vi "load csv taglist.vi"(10 "cfg file path":path) -> (2 "ok?":bool, 3 "tags":refnum<class "tag descriptor.lvclass">[](array[class]))   [LabVIEW 2013, in "PL Framework Configuration Tool.lvlib" / "EngineTags.lvclass"]
uses:
  EngineTags.lvclass
  <vilib>/NI/Tag Bus/tag/tag descriptor.lvclass
  <vilib>/NI/Tag Bus/tag/count types.vi
  <vilib>/NI/Tag Bus/tag/index to type.vi
  Robust CSV/Robust CSV.lvlib
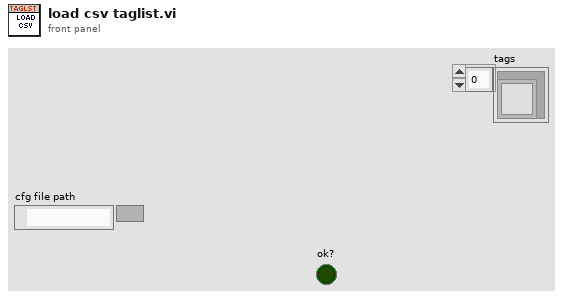
[diagram p1: front panel]
types:
  T1 = enum16{"open", "replace", "create", "open or create", "replace or create", "replace or create with confirmation"}
  T2 = typedef "tag bus.lvlib/tag descriptor.lvclass/Data Type.ctl" = enum16{"Double", "Single", "I64", "I32", "I16", "I8", "U64", "U32", "U16", "U8", "Boolean", "String", "Array of Double", "Array of Single", "Array of I64", "Array of I32", "Array of I16", "Array of I8", "Array of U64", "Array of U32", "Array of U16", "Array of U8", "Array of Boolean", "Array of String"}
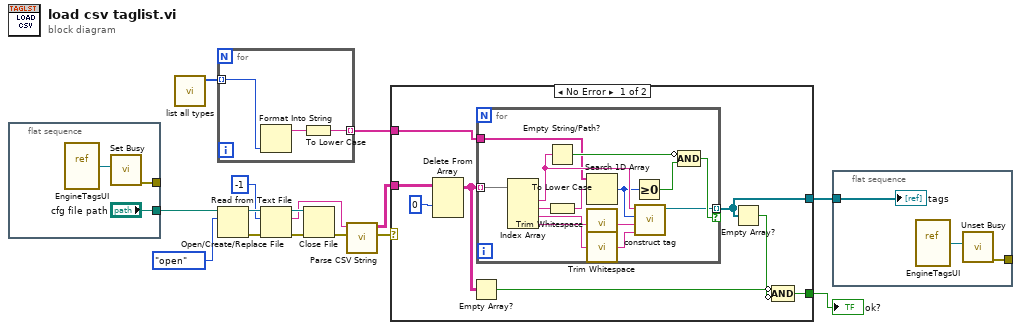
[diagram p0: block diagram]
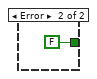
[diagram p2: hidden frame]
diagram:
  n1 = flat-sequence {
    tunnel: [w17] -> _
    tunnel: ["cfg file path"] -> w9
    frame #0 {
      n2 = vi-ref "EngineTagsUI.vi"() -> (w18:refnum<vi>)
      n3 = call <vilib>:"Set Busy.vi"("VI reference (current VI)"=w18) -> ("error out"=w17:errorcluster)  [unwired: 9 in, 1 out]
    }
  }
  n4 = call <vilib>:"list all types.vi"() -> ("all types"=w6:T2[])  [unwired: 11 in]
  n5 = for {
    tunnel: w6 -> [w21] mode=indexing
    tunnel: [w19] -> w5 mode=indexing
    n6 = Format Into String(w21) -> (resulting string=w20:string)  [unwired: 3 in, 1 out]
    n7 = To Lower Case(string=w20) -> (all lower case string=w19:string)
  }
  n8 = Open/Create/Replace File(file path (use dialog)=w9, operation (0:open)=T1."open") -> (refnum out=w13:refnum<file>, error out=w12:errorcluster)  [unwired: 4 in, 1 out]
  n9 = Read from Text File(file (use dialog)=w13, count=-1, error in=w12) -> (refnum out=w11:refnum<file>, text=w3:string, error out=w10:errorcluster)  [unwired: 1 in, 1 out]
  n10 = Close File(refnum=w11, error in=w10) -> (error out=w4:errorcluster)  [unwired: 1 out]
  n11 = call "Parse CSV String.vi"("error in"=w4, "CSV string"=w3) -> ("error out"=w1:errorcluster, "2-D array"=w2:string[][])  [unwired: 8 in]
  n12 = case shown="No Error" w1 {
    tunnel: w2 -> [w22 _]
    tunnel: [w26 _] -> w15
    tunnel: [w24 FALSE] -> w14
    tunnel: w5 -> [w23 _]
    frame No Error {
      n13 = Delete From Array(array=w22, index (row)=0) -> (array with subset deleted=w28:string[][])  [unwired: 2 in, 1 out]
      n14 = Empty Array?(array=w28) -> (empty?=w27:bool)
      n15 = for {
        tunnel: [w39] -> w26 mode=indexing if=w42
        tunnel: w28 -> [w30] mode=indexing
        tunnel: w23 -> [w33]
        n16 = Index Array(array=w30) -> (element #1=w36:string, element #2=w35:string, element #3=w37:string, element #4=w38:string)  [unwired: 4 in]
        n17 = Empty String/Path?(string/path=w36) -> (empty?=w43:bool)
        n18 = To Lower Case(string=w35) -> (all lower case string=w34:string)
        n19 = Search 1D Array(1D array=w33, element=w34) -> (index of element=w31:i32)  [unwired: 1 in]
        n20 = call <vilib>:"Trim Whitespace.vi"("string"=w38) -> ("trimmed string"=w41:string)  [unwired: 1 in]
        n21 = call <vilib>:"Trim Whitespace.vi"("string"=w37) -> ("trimmed string"=w40:string)  [unwired: 1 in]
        n22 = Greater Or Equal To 0?(x=w31) -> (x >= 0?=w32:bool)
        n23 = call <vilib>:"construct tag.vi"("raw default"=w40, "metadata"=w41, "data type"=w31, "name"=w36) -> ("system tag out"=w39:refnum<class "tag descriptor.lvclass">)  [unwired: 6 in, 1 out]
        n24 = Compound Arithmetic op=AND(invert w43, w32) -> (w42:bool)
      }
      n25 = Empty Array?(array=w26) -> (empty?=w25:bool)
      n26 = Compound Arithmetic op=AND(invert w27, invert w25) -> (w24:bool)
    }
    frame Error {
    }
  }
  "ok?" <- w14
  n27 = flat-sequence {
    tunnel: w15 -> [w45]
    tunnel: [w46] -> _
    frame #0 {
      n28 = vi-ref "EngineTagsUI.vi"() -> (w47:refnum<vi>)
      n29 = call <vilib>:"Unset Busy.vi"("VI reference (current VI)"=w47) -> ("error out"=w46:errorcluster)  [unwired: 10 in]
      "tags" <- w45
    }
  }
